vi "Config Type.vi"(11 "Stop Log Command in":refnum<class "Stop Log Command.lvclass">) -> (2 "Command Config Type":refnum<class "Command Config.lvclass">)   [LabVIEW 2020, in "VolatusSeq.lvlib" / "Stop Log Command.lvclass"]
uses:
  Stop Log Command.lvclass
  Stop Log Command.lvclass/Stop Log Command.ctl
  VolatusSeqConfig/Stop Log Command Config/Stop Log Command Config.lvclass
  C:/dev/lv20CE/relink/lv-volatus/VolatusSeqConfig/Command Config/Command Config.lvclass
  C:/dev/lv20CE/relink/lv-volatus/VolatusSeqConfig/Stop Log Command Config/Stop Log Command Config.lvclass
  VolatusSeqConfig/Command Config/Command Config.lvclass
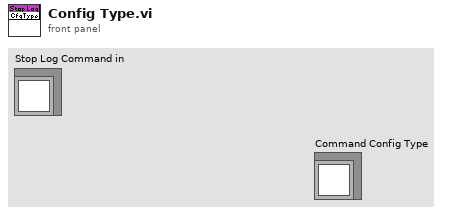
[diagram p1: front panel]
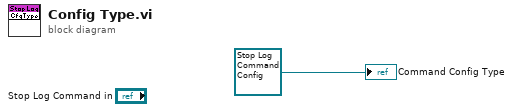
[diagram p0: block diagram]
diagram:
  "Command Config Type" <- refnum<class "Stop Log Command Config.lvclass"> refnum ("VolatusSeqConfig.lvlib:Stop Log Command Config.lvclass")
